vi "Polar To Complex - RM,RM.vi"(1 "Argument Q":T1, 2 "Modulus r":T1) -> (0 "Complex Matrix r*e^iQ":T2)   [LabVIEW 2017, in "NI_Matrix.lvlib"]
doc: "Creates a complex number from two values in polar notation."
uses:
  NI_Matrix.lvlib
  RealMatrix.ctl
  ComplexMatrix.ctl
  Array To Matrix - CA2.vi
  Matrix To Array - RM.vi
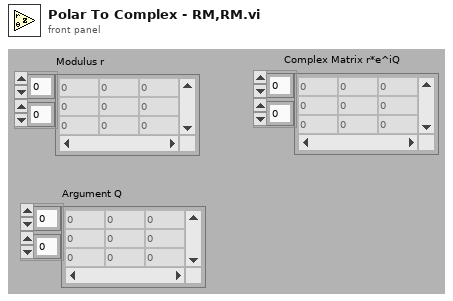
[diagram p1: front panel]
types:
  T1 = typedef "NI_Matrix.lvlib/RealMatrix.ctl" = dbl[][]
  T2 = typedef "NI_Matrix.lvlib/ComplexMatrix.ctl" = cdb[][]
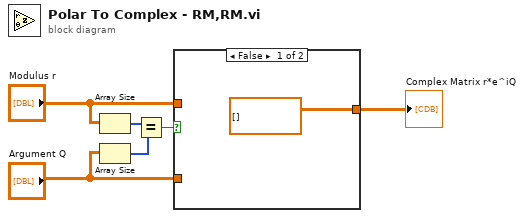
[diagram p0: block diagram]
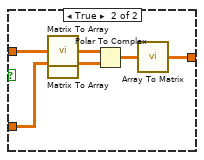
[diagram p2: hidden frame]
diagram:
  n1 = Array Size(array="Modulus r") -> (size(s)=w5:i32[])
  n2 = Array Size(array="Argument Q") -> (size(s)=w6:i32[])
  n3 = Equal?(x=w5, y=w6) -> (x = y?=w4:bool)
  n4 = case shown="False" w4 {
    tunnel: "Modulus r" -> [_ w12]
    tunnel: "Argument Q" -> [_ w10]
    tunnel: [T2 [] ("R + Ii") w8] -> w1
    frame False {
    }
    frame True {
      n5 = call-poly "Matrix To Array.vi"("Real Matrix"=w12) -> ("Real 2D Array"=w13:dbl[][])
      n6 = call-poly "Matrix To Array.vi"("Real Matrix"=w10) -> ("Real 2D Array"=w11:dbl[][])
      n7 = Polar To Complex(1:w11, 2:w13) -> (0:w9:cdb[][])
      n8 = call-poly "Array To Matrix.vi"("Complex 2D Array"=w9) -> ("Complex Matrix"=w8:T2)
    }
  }
  "Complex Matrix r*e^iQ" <- w1
